vi "Lab4(II).vi"() -> ()   [LabVIEW 2021]
panel:
  out "7":bool
  out "6":bool
  out "3":bool
  out "5":bool
  out "4":bool
  out "2":bool
  out "1":bool
  in  "Number":dbl
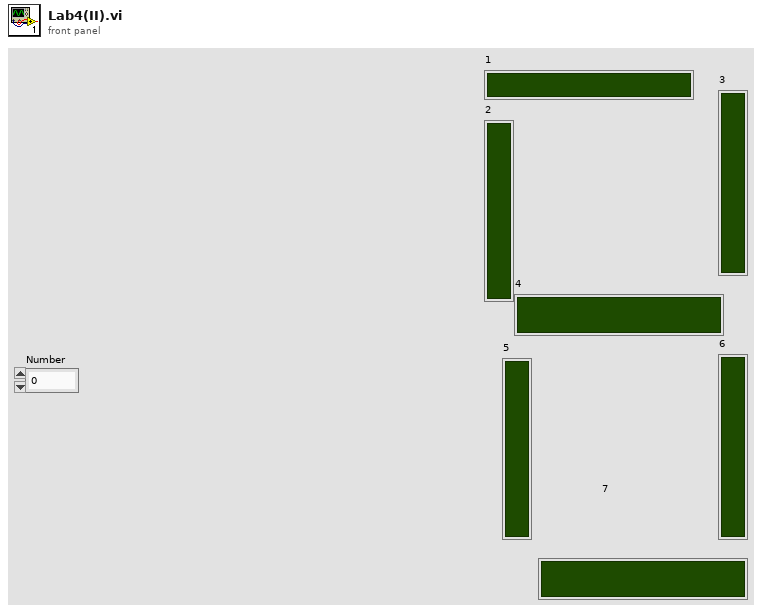
[diagram p1: front panel]
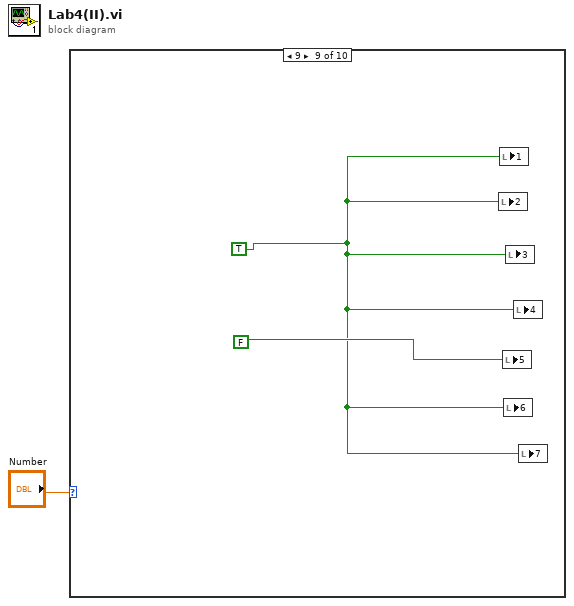
[diagram p0: block diagram]
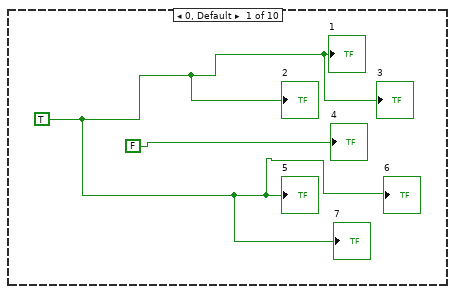
[diagram p2: hidden frame]
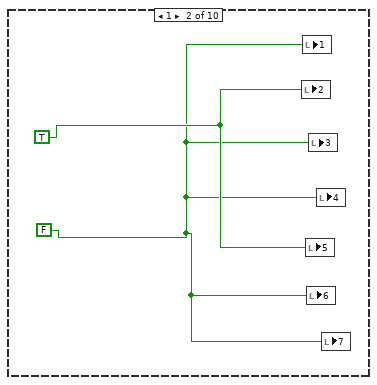
[diagram p3: hidden frame]
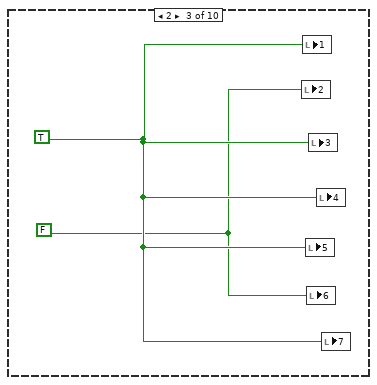
[diagram p4: hidden frame]
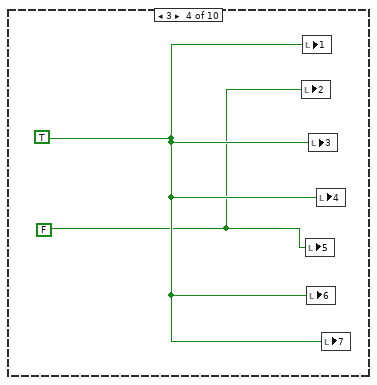
[diagram p5: hidden frame]
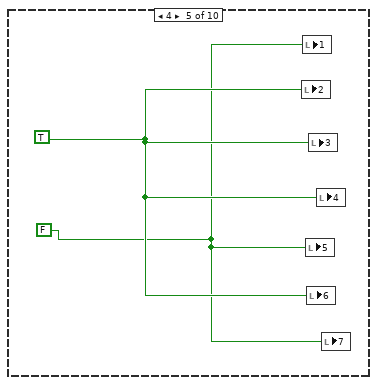
[diagram p6: hidden frame]
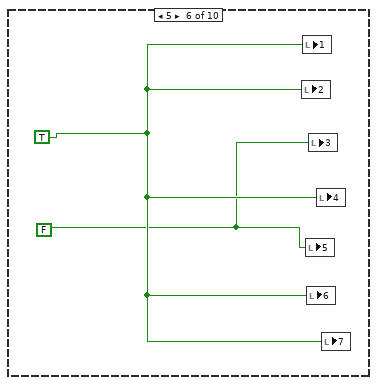
[diagram p7: hidden frame]
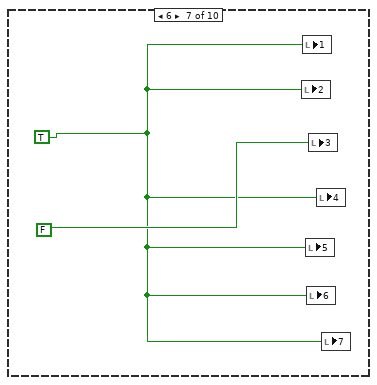
[diagram p8: hidden frame]
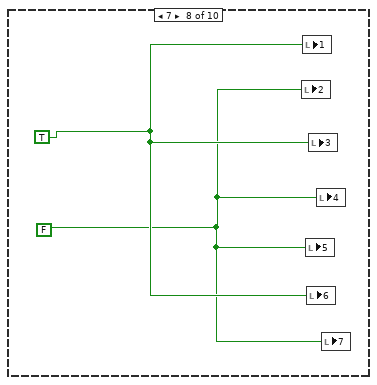
[diagram p9: hidden frame]
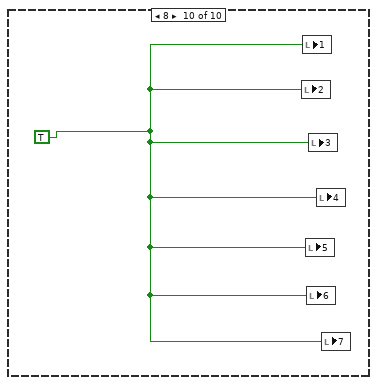
[diagram p10: hidden frame]
diagram:
  n1 = case shown="9" "Number" {
    frame 0, Default {
      w2 = TRUE
      "1" <- w2
      "2" <- w2
      "4" <- FALSE
      "5" <- w2
      "3" <- w2
      "6" <- w2
      "7" <- w2
    }
    frame 1 {
      w5 = TRUE
      w4 = FALSE
      n2 = local write "2"(w5) -> ()
      n3 = local write "1"(w4) -> ()
      n4 = local write "5"(w5) -> ()
      n5 = local write "6"(w4) -> ()
      n6 = local write "3"(w4) -> ()
      n7 = local write "4"(w4) -> ()
      n8 = local write "7"(w4) -> ()
    }
    frame 2 {
      w7 = TRUE
      w6 = FALSE
      n9 = local write "2"(w6) -> ()
      n10 = local write "1"(w7) -> ()
      n11 = local write "5"(w7) -> ()
      n12 = local write "6"(w6) -> ()
      n13 = local write "3"(w7) -> ()
      n14 = local write "4"(w7) -> ()
      n15 = local write "7"(w7) -> ()
    }
    frame 3 {
      w9 = TRUE
      w8 = FALSE
      n16 = local write "2"(w8) -> ()
      n17 = local write "1"(w9) -> ()
      n18 = local write "5"(w8) -> ()
      n19 = local write "6"(w9) -> ()
      n20 = local write "3"(w9) -> ()
      n21 = local write "4"(w9) -> ()
      n22 = local write "7"(w9) -> ()
    }
    frame 4 {
      w11 = TRUE
      w10 = FALSE
      n23 = local write "2"(w11) -> ()
      n24 = local write "1"(w10) -> ()
      n25 = local write "5"(w10) -> ()
      n26 = local write "6"(w11) -> ()
      n27 = local write "3"(w11) -> ()
      n28 = local write "4"(w11) -> ()
      n29 = local write "7"(w10) -> ()
    }
    frame 5 {
      w13 = TRUE
      w12 = FALSE
      n30 = local write "2"(w13) -> ()
      n31 = local write "1"(w13) -> ()
      n32 = local write "5"(w12) -> ()
      n33 = local write "6"(w13) -> ()
      n34 = local write "3"(w12) -> ()
      n35 = local write "4"(w13) -> ()
      n36 = local write "7"(w13) -> ()
    }
    frame 6 {
      w14 = TRUE
      n37 = local write "2"(w14) -> ()
      n38 = local write "1"(w14) -> ()
      n39 = local write "5"(w14) -> ()
      n40 = local write "6"(w14) -> ()
      n41 = local write "3"(FALSE) -> ()
      n42 = local write "4"(w14) -> ()
      n43 = local write "7"(w14) -> ()
    }
    frame 7 {
      w17 = TRUE
      w16 = FALSE
      n44 = local write "2"(w16) -> ()
      n45 = local write "1"(w17) -> ()
      n46 = local write "5"(w16) -> ()
      n47 = local write "6"(w17) -> ()
      n48 = local write "3"(w17) -> ()
      n49 = local write "4"(w16) -> ()
      n50 = local write "7"(w16) -> ()
    }
    frame 9 {
      w18 = TRUE
      n51 = local write "2"(w18) -> ()
      n52 = local write "1"(w18) -> ()
      n53 = local write "5"(FALSE) -> ()
      n54 = local write "6"(w18) -> ()
      n55 = local write "3"(w18) -> ()
      n56 = local write "4"(w18) -> ()
      n57 = local write "7"(w18) -> ()
    }
    frame 8 {
      w20 = TRUE
      n58 = local write "2"(w20) -> ()
      n59 = local write "1"(w20) -> ()
      n60 = local write "5"(w20) -> ()
      n61 = local write "6"(w20) -> ()
      n62 = local write "3"(w20) -> ()
      n63 = local write "4"(w20) -> ()
      n64 = local write "7"(w20) -> ()
    }
  }
